vi "Write Iteration.vi"(8 "error in (no error)":errorcluster, 10 "Iteration":refnum<vi>, 11 "Measurement in":refnum<class "Measurement.lvclass">) -> (0 "error out":errorcluster, 3 "Measurement out":refnum<class "Measurement.lvclass">)   [LabVIEW 2016, in "Measurement Actor.lvlib" / "Measurement.lvclass"]
uses:
  Measurement.lvclass
  Measurement.lvclass/Measurement.ctl
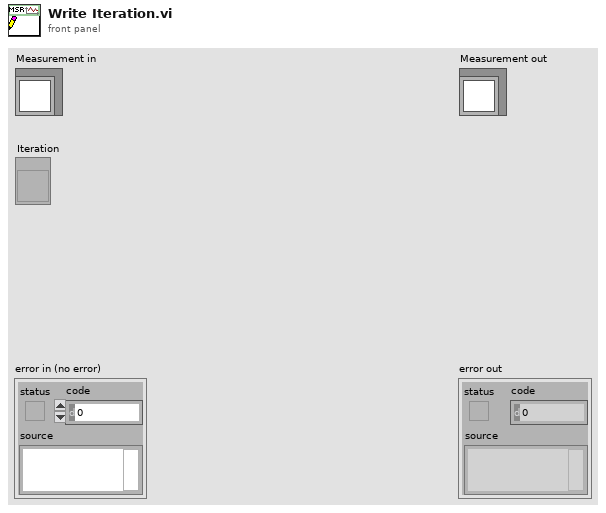
[diagram p1: front panel]
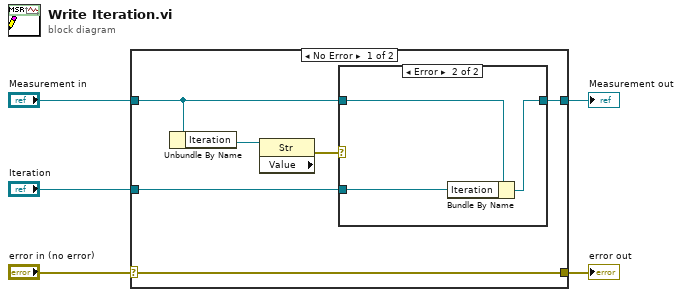
[diagram p0: block diagram]
diagram:
  n1 = case shown="No Error" "error in (no error)" {
    selector: "error in (no error)" -> [w11 w16]
    tunnel: [w11 w16] -> w4
    tunnel: [w10 w17] -> w2
    tunnel: "Measurement in" -> [w8 w17]
    tunnel: "Iteration" -> [w9 _]
    frame No Error {
      n2 = Unbundle By Name(w8) -> ("Iteration"=w7:refnum<vi>)
      n3 = property class="Str" props=["Value"](reference=w7) -> (error out=w6:errorcluster)  [unwired: 1 in, 2 out]
      n4 = case shown="Error" w6 {
        tunnel: [w12 w15] -> w10
        tunnel: w9 -> [_ w14]
        tunnel: w8 -> [w12 w13]
        frame No Error {
        }
        frame Error {
          n5 = Bundle By Name(cluster=w13, "Iteration"=w14) -> (w15:refnum<class "Measurement.lvclass">)
        }
      }
    }
    frame Error {
    }
  }
  "error out" <- w4
  "Measurement out" <- w2
